vi "RS485 Read Rotork FPGA-2.vi"() -> (2 "Valve position":u8[](array[numeric]))   [LabVIEW 2014]
uses:
  <vilib>/rvi/eio/common/nirviEmuTemplateMethod_errors.vi
  <vilib>/eio/EIOMethodNode/EIOMethodNode.xnode
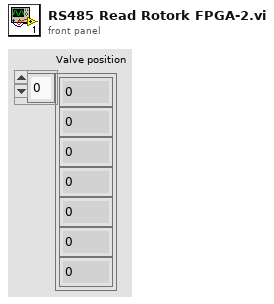
[diagram p1: front panel]
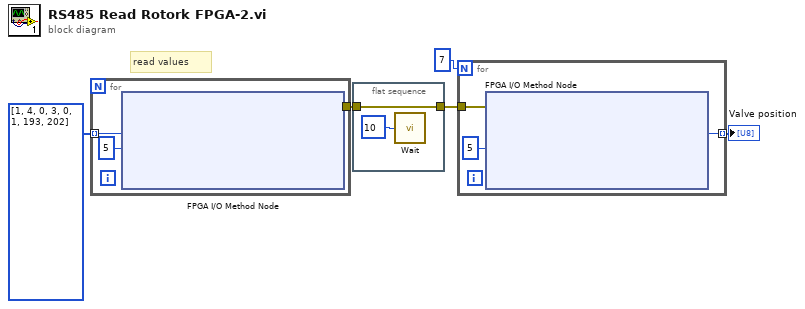
[diagram p0: block diagram]
diagram:
  # "read values"
  n1 = for {
    tunnel: u8[] [1, 4, 0, 3, 0, 1, 193, 202] ("appended array") -> [w8] mode=indexing
    tunnel: [w6] -> w4
    n2 = xnode "FPGA I/O Method Node"("Data"=w8, "Timeout (ms)"=5) -> ("error out"=w6:errorcluster)  [unwired: 2 in, 2 out]
  }
  n3 = flat-sequence {
    tunnel: w4 -> [w9]
    tunnel: [w9] -> w3
    frame #0 {
      n4 = call "Wait"("Count(mSec)"=u32 10) -> ()  [unwired: 1 out]
    }
  }
  n5 = for {
    N: 7 -> [_]
    tunnel: w3 -> [w13]
    tunnel: [w12] -> w2 mode=indexing
    n6 = xnode "FPGA I/O Method Node"("error in"=w13, "Timeout (ms)"=5) -> ("Data"=w12:u8)  [unwired: 1 in, 3 out]
  }
  "Valve position" <- w2
